vi "Add Date Yields.vi"(8 "error in (no error)":errorcluster, 10 "Cluster":T1, 11 "Master in":refnum<class "Master.lvclass">) -> (0 "error out":errorcluster, 3 "Master out":refnum<class "Master.lvclass">)   [LabVIEW 2014, in "Master.lvclass"]
uses:
  Master/Master.lvclass
  Master/Master.lvclass/Master.ctl
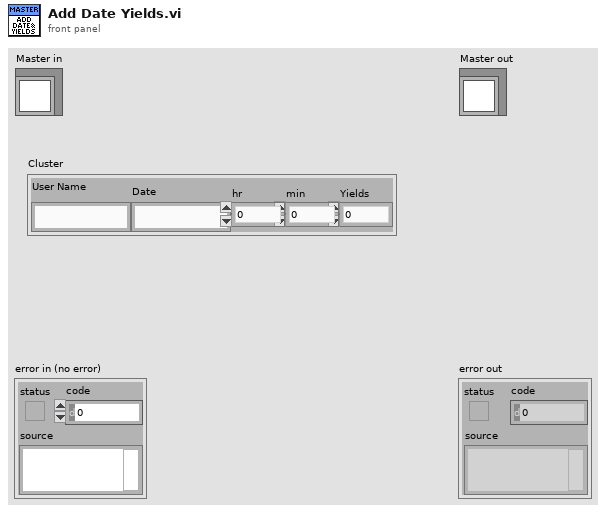
[diagram p1: front panel]
types:
  T1 = cluster{"User Name":string, "Date":string, "Yields":dbl, "min":dbl, "hr":dbl}
  T2 = cluster{"Production Record":cluster{"User":string, "Date":string, "Yields":dbl, "hour":i32, "minute":i32}[], "Total Yields":dbl}
  T3 = cluster{"User":string, "Date":string, "Yields":dbl, "hour":i32, "minute":i32}[]
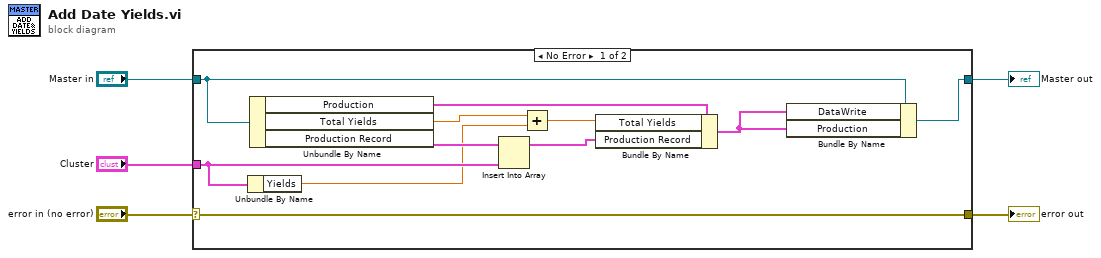
[diagram p0: block diagram]
diagram:
  n1 = case shown="No Error" "error in (no error)" {
    selector: "error in (no error)" -> [w16 w18]
    tunnel: [w16 w18] -> w4
    tunnel: [w13 w17] -> w2
    tunnel: "Master in" -> [w14 w17]
    tunnel: "Cluster" -> [w12 _]
    frame No Error {
      n2 = Unbundle By Name(w12) -> ("Yields"=w10:dbl)
      n3 = Unbundle By Name(w14) -> ("Production"=w9:T2, "Total Yields"=w11:dbl, "Production Record"=w15:T3)
      n4 = Insert Into Array(array=w15, new element=w12) -> (w7:T3)  [unwired: 1 in]
      n5 = Add(x=w11, y=w10) -> (x+y=w8:dbl)
      n6 = Bundle By Name(cluster=w9, "Total Yields"=w8, "Production Record"=w7) -> (w6:T2)
      n7 = Bundle By Name(cluster=w14, "DataWrite"=w6, "Production"=w6) -> (w13:refnum<class "Master.lvclass">)
    }
    frame Error {
    }
  }
  "error out" <- w4
  "Master out" <- w2
